vi "Channel_Number.vi"(7 "Main Cluster IN":T1) -> (0 "Total Number of Channels on Drop 1":i32, 1 "Total Number of Channels on Drop 0":i32, 2 "Total Number of Channels":i32)   [LabVIEW 2016]
uses:
  Control/Control_Main.ctl
  Control/Control_ModuleArray.ctl
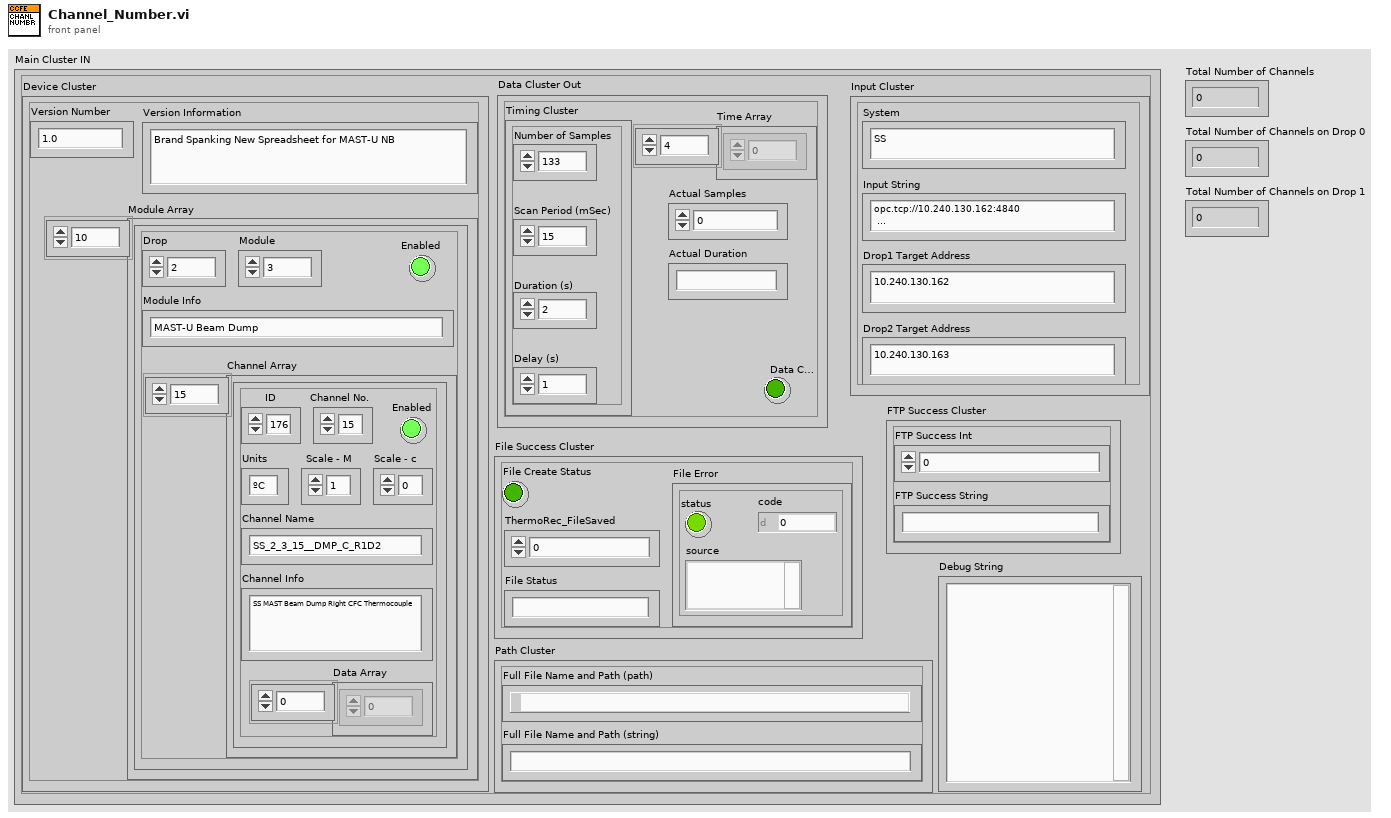
[diagram p1: front panel]
types:
  T1 = typedef "Control_Main.ctl" = cluster{"Device Cluster":cluster{"Module Array":T2, "Version Number":string, "Version Information":string}, "Input Cluster":cluster{"Input String":string, "Drop1 Target Address":string, "Drop2 Target Address":string, "System":string}, "Data Cluster Out":cluster{"Timing Cluster":cluster{"Number of Samples":i32, "Scan Period (mSec)":u32, "Duration (s)":dbl, "Delay (s)":dbl}, "Time Array":dbl[], "Actual Samples":i32, "Actual Duration":string, "Data Collection Error":bool}, "Path Cluster":cluster{"Full File Name and Path (path)":path, "Full File Name and Path (string)":string}, "File Success Cluster":cluster{"ThermoRec_FileSaved":i32, "File Create Status":bool, "File Error":errorcluster, "File Status":string}, "FTP Success Cluster":cluster{"FTP Success Int":i32, "FTP Success String":string}, "Debug String":string}
  T2 = typedef "Control_ModuleArray.ctl" = cluster{"Drop":i32, "Module":i32, "Module Info":string, "Enabled":bool, "Channel Array":cluster{"ID":i32, "Channel No.":i32, "Enabled":bool, "Channel Name":string, "Channel Info":string, "Units":string, "Scale - M":dbl, "Scale - c":dbl, "Data Array":dbl[]}[]}[]
  T3 = cluster{"ID":i32, "Channel No.":i32, "Enabled":bool, "Channel Name":string, "Channel Info":string, "Units":string, "Scale - M":dbl, "Scale - c":dbl, "Data Array":dbl[]}[]
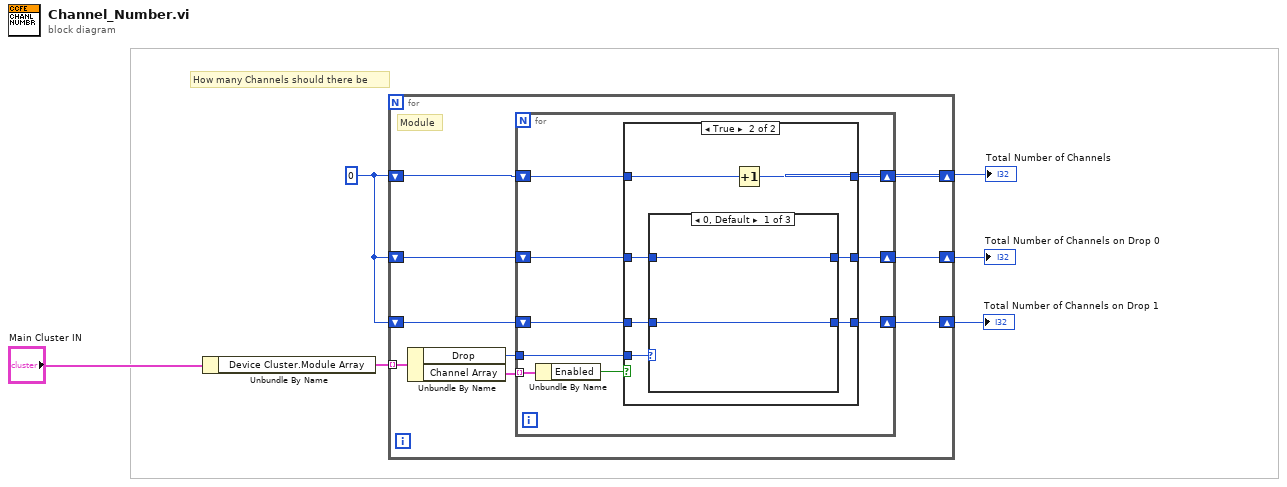
[diagram p0: block diagram]
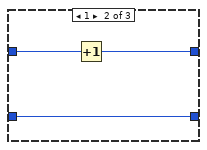
[diagram p3: hidden frame]
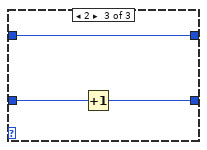
[diagram p4: hidden frame]
diagram:
  w3 = 0
  # "How many Channels should there be"
  n1 = Unbundle By Name("Main Cluster IN") -> ("Device Cluster.Module Array"=w6:T2)
  n2 = for {
    tunnel: w6 -> [w15] mode=indexing
    shift-right: [w13] -> w4
    shift-left: w3 -> [w12]
    shift-right: [w9] -> w2
    shift-left: w3 -> [w10]
    shift-right: [w7] -> w1
    shift-left: w3 -> [w8]
    # "Module"
    n3 = Unbundle By Name(w15) -> ("Drop"=w11:i32, "Channel Array"=w14:T3)
    n4 = for {
      tunnel: w14 -> [w24] mode=indexing
      shift-right: [w21] -> w13
      shift-left: w12 -> [w22]
      tunnel: w11 -> [w20]
      shift-right: [w18] -> w9
      shift-left: w10 -> [w19]
      shift-right: [w16] -> w7
      shift-left: w8 -> [w17]
      n5 = Unbundle By Name(w24) -> ("Enabled"=w23:bool)
      n6 = case shown="True" w23 {
        tunnel: w22 -> [w27 w33]
        tunnel: [w27 w34] -> w21
        tunnel: w20 -> [_ w32]
        tunnel: [w26 w30] -> w18
        tunnel: w19 -> [w26 w31]
        tunnel: w17 -> [w25 w29]
        tunnel: [w25 w28] -> w16
        frame False {
        }
        frame True {
          n7 = case shown="0, Default" w32 {
            tunnel: w31 -> [w35 w39 w42]
            tunnel: [w35 w38 w42] -> w30
            tunnel: w29 -> [w36 w37 w41]
            tunnel: [w36 w37 w40] -> w28
            frame 0, Default {
            }
            frame 1 {
              n8 = Increment(x=w39) -> (x+1=w38:i32)
            }
            frame 2 {
              n9 = Increment(x=w41) -> (x+1=w40:i32)
            }
          }
          n10 = Increment(x=w33) -> (x+1=w34:i32)
        }
      }
    }
  }
  "Total Number of Channels on Drop 1" <- w1
  "Total Number of Channels on Drop 0" <- w2
  "Total Number of Channels" <- w4
